vi "readI32.vi"(8 "error in (no error)":errorcluster, 11 "ModbusBuffer in":refnum<class "ModbusBuffer.lvclass">) -> (0 "error out":errorcluster, 2 "Output":i32, 3 "ModbusBuffer out":refnum<class "ModbusBuffer.lvclass">)   [LabVIEW 2016, in "RTModbus.lvlib" / "ModbusBuffer.lvclass"]
uses:
  ModbusBuffer.lvclass
  ModbusBuffer.lvclass/ModbusBuffer.ctl
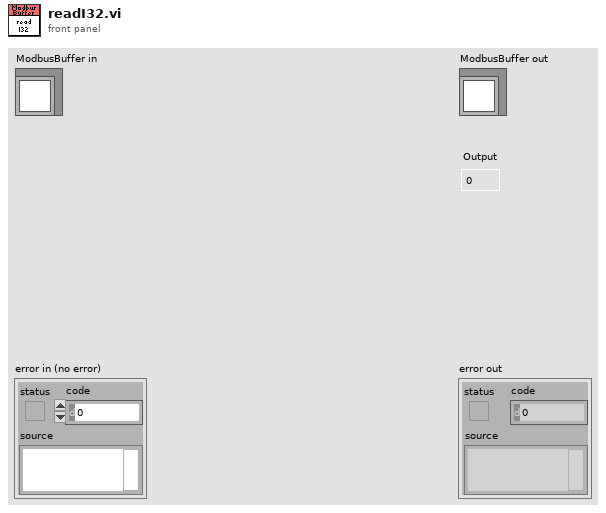
[diagram p1: front panel]
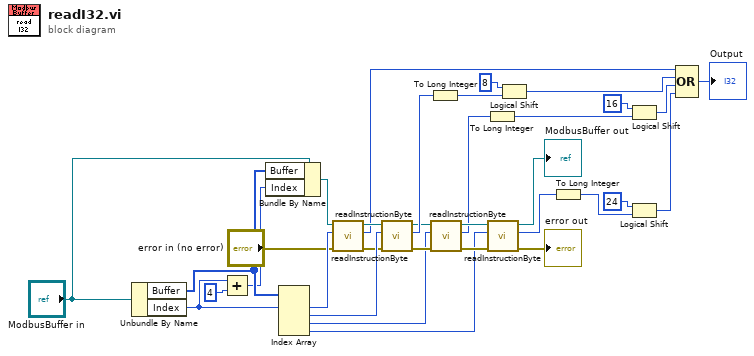
[diagram p0: block diagram]
diagram:
  n1 = Unbundle By Name("ModbusBuffer in") -> ("Buffer"=w32:u16[], "Index"=w28:i32)
  n2 = Add(x=w28, y=4) -> (x+y=w26:i32)
  n3 = Bundle By Name(cluster="ModbusBuffer in", "Buffer"=w32, "Index"=w26) -> (w30:refnum<class "ModbusBuffer.lvclass">)
  n4 = Index Array(array=w32, index #1=w28) -> (element #1=w31:u16, element #2=w24:u16, element #3=w2:u16, element #4=w1:u16)  [unwired: 3 in]
  n5 = call "readInstructionByte.vi"("error in (no error)"="error in (no error)", "Instruction"=w31, "ModbusBuffer in"=w30) -> ("error out"=w22:errorcluster, "Output"=w23:u8, "ModbusBuffer out"=w25:refnum<class "ModbusBuffer.lvclass">)  [unwired: 6 in]
  n6 = call "readInstructionByte.vi"("error in (no error)"=w22, "Instruction"=w24, "ModbusBuffer in"=w25) -> ("error out"=w13:errorcluster, "Output"=w18:u8, "ModbusBuffer out"=w16:refnum<class "ModbusBuffer.lvclass">)  [unwired: 6 in]
  n7 = To Long Integer(number=w18) -> (32bit integer=w17:i32)
  n8 = call "readInstructionByte.vi"("error in (no error)"=w13, "Instruction"=w2, "ModbusBuffer in"=w16) -> ("error out"=w12:errorcluster, "Output"=w6:u8, "ModbusBuffer out"=w15:refnum<class "ModbusBuffer.lvclass">)  [unwired: 6 in]
  n9 = To Long Integer(number=w6) -> (32bit integer=w10:i32)
  n10 = call "readInstructionByte.vi"("error in (no error)"=w12, "Instruction"=w1, "ModbusBuffer in"=w15) -> ("error out"=→"error out":errorcluster, "Output"=w5:u8, "ModbusBuffer out"=→"ModbusBuffer out":refnum<class "ModbusBuffer.lvclass">)  [unwired: 6 in]
  n11 = Logical Shift(y=i16 8, x=w17) -> (x << y=w20:i32)
  n12 = To Long Integer(number=w5) -> (32bit integer=w7:i32)
  n13 = Logical Shift(y=i16 16, x=w10) -> (x << y=w3:i32)
  n14 = Logical Shift(y=i16 24, x=w7) -> (x << y=w4:i32)
  n15 = Compound Arithmetic op=OR(w23, w20, w3, w4) -> (→"Output":i32)
